vi "ma_manage resamp timing single-shot.vi"(0 "waveform in":waveform(dbl), 1 "open interval? (T)":bool=TRUE, 2 "closed interval asymmetric":bool=TRUE, 5 "dt":dbl=1.0 format="%.2p", 7 "state info in":cluster{"buffer":dbl[], "t0 history":timestamp} {"t0 history" format="%<%.4X>T"; "buffer" format="%.2p"}, 11 "error in":errorcluster) -> (4 "waveform to be processed":waveform(dbl), 6 "#elements":i32, 10 "used t0":timestamp format="%<%.4X>T", 14 "t0 adjusted warning":bool, 15 "error out":errorcluster)   [LabVIEW 2020, in "NI_MAPro.lvlib"]
doc: "This VI re-samples an unevenly sampled input signal to an evenly sampled waveform according to specified t0 and dt. If the specified t0 value is less than the first value of input X-array (that is the timestamp of the first input sample), then the VI will coerce t0 to the first valid value (greater than X(0)) that also fulfill the relation:\n\nT0_adjusted - t0_in = n * dt_in\n\nThis guarranty that any later comparison of waveforms will be correct with repsect to absolute time."
uses:
  NI_MAPro.lvlib
panel:
  # "open"
  # "closed"
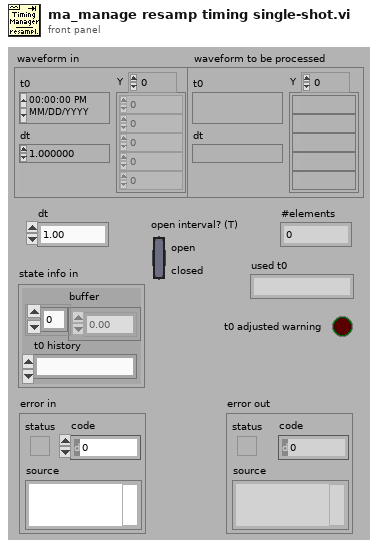
[diagram p1: front panel]
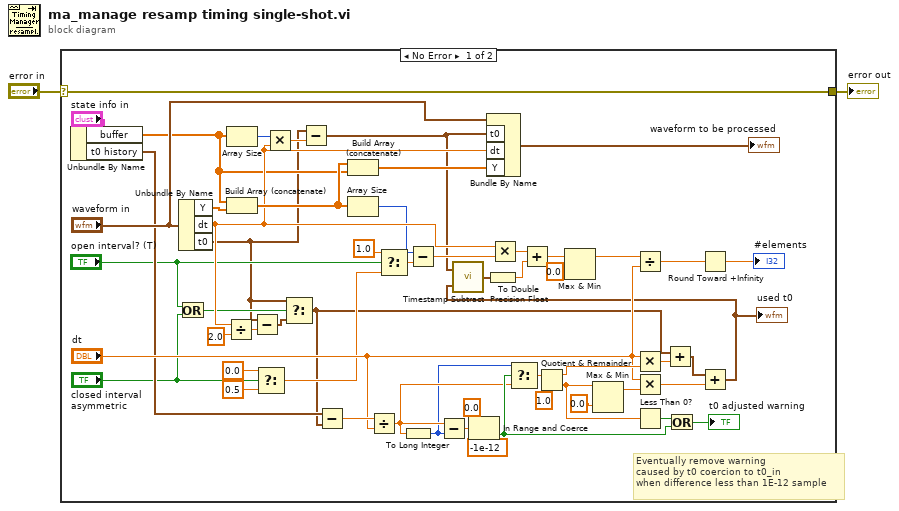
[diagram p0: block diagram]
diagram:
  n1 = case shown="No Error" "error in" {
    selector: "error in" -> [w19 w59]
    tunnel: [w19 w59] -> w2
    frame No Error {
      # "Eventually remove warning\ncaused by t0 coercion to t0_in\nwhen difference less than 1E-12 sample"
      n2 = Unbundle By Name("state info in") -> ("buffer"=w23:dbl[], "t0 history"=w24:timestamp)
      n3 = Or(x="open interval? (T)", y="closed interval asymmetric") -> (x .or. y?=w16:bool)
      n4 = Unbundle By Name("waveform in") -> ("Y"=w48:dbl[], "dt"=w33:dbl, "t0"=w6:timestamp)
      n5 = Divide(x=w33, y=2.0) -> (x/y=w37:dbl)
      n6 = Array Size(array=w23) -> (size(s)=w52:i32)
      n7 = Build Array (concatenate)(w23, w48) -> (w38:dbl[])
      n8 = Subtract(x=w6, y=w37) -> (x-y=w17:timestamp)
      n9 = Select(t=0.0 ("f"), s="closed interval asymmetric", f=0.5) -> (s? t:f=w11:dbl)
      n10 = Multiply(x=w52, y=w33) -> (x*y=w51:dbl)
      n11 = Select(t=w6, s=w16, f=w17) -> (s? t:f=w7:timestamp)
      n12 = Subtract(x=w6, y=w51) -> (x-y=w5:timestamp)
      n13 = Subtract(x=w24, y=w7) -> (x-y=w57:dbl)
      n14 = Build Array (concatenate)(w38, w23) -> (w39:dbl[])
      n15 = Array Size(array=w38) -> (size(s)=w31:i32)
      n16 = Divide(x=w57, y="dt") -> (x/y=w22:dbl)
      n17 = Select(t=1.0, s="open interval? (T)", f=w11) -> (s? t:f=w32:dbl)
      n18 = To Long Integer(number=w22) -> (32bit integer=w20:i32)
      n19 = Subtract(x=w31, y=w32) -> (x-y=w30:dbl)
      n20 = Subtract(x=w22, y=w20) -> (x-y=w21:dbl)
      n21 = In Range and Coerce(upper limit=0.0, x=w21, lower limit=-1e-12) -> (In Range?=w41:bool)  [unwired: 1 out]
      n22 = Bundle By Name(cluster="waveform in", "t0"=w5, "dt"=w33, "Y"=w39) -> (→"waveform to be processed":waveform(dbl))
      n23 = Multiply(x=w33, y=w30) -> (x*y=w47:dbl)
      n24 = Select(t=w20, s=w41, f=w22) -> (s? t:f=w43:dbl)
      n25 = Quotient & Remainder(x=w43, y=1.0) -> (x-y*floor(x/y)=w46:dbl, floor(x/y)=w54:dbl)
      n26 = Max & Min(x=w54, y=0.0) -> (max(x,y)=w56:dbl)  [unwired: 1 out]
      n27 = Multiply(x="dt", y=w46) -> (x*y=w9:dbl)
      n28 = Multiply(x="dt", y=w56) -> (x*y=w8:dbl)
      n29 = Less Than 0?(x=w54) -> (x < 0?=w42:bool)
      n30 = Add(x=w7, y=w9) -> (x+y=w10:timestamp)
      n31 = Or(x=w42, y=w41) -> (x .or. y?=→"t0 adjusted warning":bool)
      n32 = Add(x=w10, y=w8) -> (x+y=w4:timestamp)
      "used t0" <- w4
      n33 = call "Timestamp Subtract.vi"("y"=w4, "x"=w5) -> ("x - y"=w53:timestamp)
      n34 = To Double Precision Float(number=w53) -> (double precision float=w3:dbl)
      n35 = Add(x=w47, y=w3) -> (x+y=w35:dbl)
      n36 = Max & Min(x=w35, y=0.0) -> (max(x,y)=w49:dbl)  [unwired: 1 out]
      n37 = Divide(x=w49, y="dt") -> (x/y=w34:dbl)
      n38 = Round Toward +Infinity(x=w34) -> (ceil(x): smallest int >= x=→"#elements":dbl)
    }
    frame Error {
    }
  }
  "error out" <- w2
